vi "Device Errors.vi"(8 "error in (no error)":errorcluster, 11 "VisaComms in":refnum<class "VisaComms.lvclass">) -> (0 "error out":errorcluster, 3 "VisaComms out":refnum<class "VisaComms.lvclass">)   [LabVIEW 2020, in "CTI.lvlib" / "VisaComms.lvclass"]
uses:
  VisaComms.lvclass
  VisaComms.lvclass/VisaComms.ctl
  Clean Visa Errors.vi
  CTI.lvlib
panel:
  out "Buffers":string[](array[string])
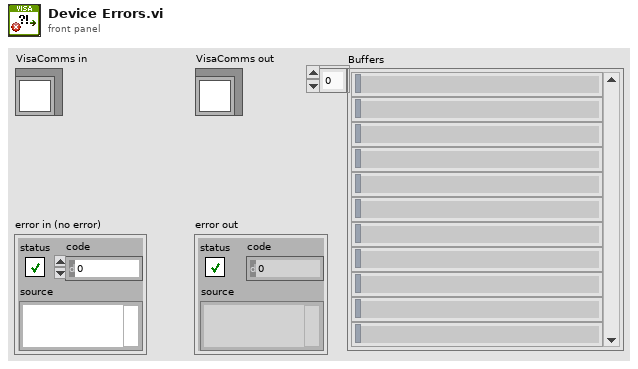
[diagram p1: front panel]
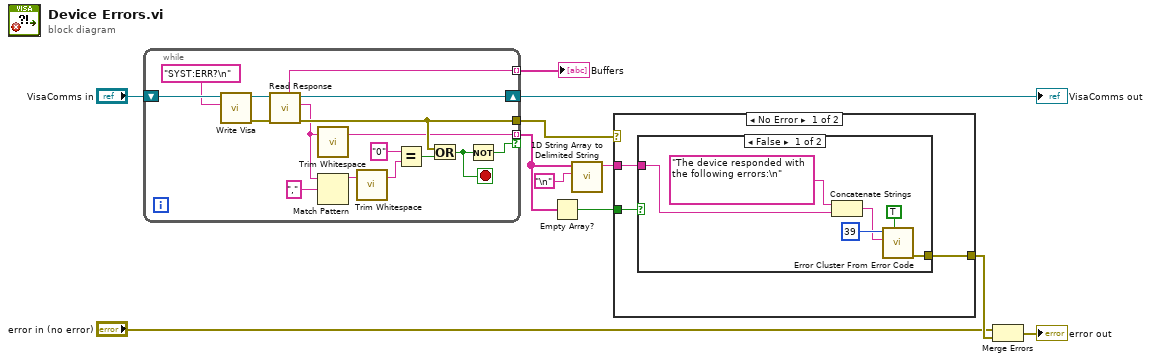
[diagram p0: block diagram]
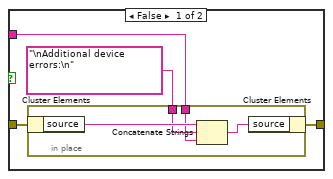
[diagram p4: hidden frame]
diagram:
  n1 = while {
    shift-right: [w17] -> w10
    shift-left: "VisaComms in" -> [w27]
    tunnel: [w18] -> w9
    tunnel: [w13] -> w7 mode=indexing if=w15
    tunnel: [w12] -> w1 mode=indexing
    stop <- w16 stop-if-true
    n2 = call "Write Visa.vi"("write buffer"="SYST:ERR?\n", "VisaComms in"=w27) -> ("error out"=w24:errorcluster, "VisaComms out"=w25:refnum<class "VisaComms.lvclass">)  [unwired: 7 in, 1 out]
    n3 = call "Read Response.vi"("error in (no error)"=w24, "VisaComms in"=w25) -> ("error out"=w18:errorcluster, "Response"=w14:string, "VisaComms out"=w17:refnum<class "VisaComms.lvclass">, "Buffer"=w12:string)  [unwired: 6 in]
    n4 = call "Trim Whitespace.vi"("String in"=w14) -> ("Trimmed"=w13:string)  [unwired: 2 in]
    n5 = Match Pattern(string=w14, regular expression=",") -> (before substring=w22:string)  [unwired: 1 in, 3 out]
    n6 = call "Trim Whitespace.vi"("String in"=w22) -> ("Trimmed"=w21:string)  [unwired: 2 in]
    n7 = Equal?(x="0", y=w21) -> (x = y?=w19:bool)
    n8 = Or(x=w18, y=w19) -> (x .or. y?=w16:bool)
    n9 = Not(x=w16) -> (.not. x?=w15:bool)
  }
  "VisaComms out" <- w10
  "Buffers" <- w1
  n10 = Empty Array?(array=w7) -> (empty?=w8:bool)
  n11 = call <vilib>:"1D String Array to Delimited String.vi"("delimiter"="\n", "string array"=w7) -> ("delimited string"=w5:string)  [unwired: 9 in]
  n12 = case shown="No Error" w9 {
    selector: w9 -> [_ w40]
    tunnel: w5 -> [w30 w38]
    tunnel: w8 -> [w29 w39]
    tunnel: [w28 w37] -> w4
    frame No Error {
      n13 = case shown="False" w29 {
        tunnel: w30 -> [w32 _]
        tunnel: [w31 _] -> w28
        frame False {
          n14 = Concatenate Strings("The device responded with the following errors:\n", w32) -> (w33:string)
          n15 = call <vilib>:"Error Cluster From Error Code.vi"("show call chain? (False)"=TRUE, "error message (\"\")"=w33, "error code (0)"=39) -> ("error out"=w31:errorcluster)  [unwired: 6 in]
        }
        frame True {
          # "No errors"
        }
      }
    }
    frame Error {
      n16 = case shown="True" w39 {
        tunnel: w38 -> [w42 _]
        tunnel: w40 -> [w44 w49]
        tunnel: [w41 w49] -> w37
        frame False {
          n17 = in-place {
            in-place-border: "\nAdditional device errors:\n" -> [w47]
            in-place-border: w42 -> [w46]
            n18 = in-place-cluster #1(w44) -> ("source"=w48:string)
            n19 = Concatenate Strings(w48, w47, w46) -> (w45:string)
            n20 = in-place-cluster #1("source"=w45) -> (w41:errorcluster)
          }
        }
        frame True {
        }
      }
    }
  }
  n21 = Merge Errors("error in (no error)", w4) -> (→"error out":errorcluster)
